vi "Query Chan Parameters (Input).vi"(7 "Channel (1: Chan A)":i32(ring)=1 items=["Channel A"=1, "Channel B"=2, "Channel C"=3, "Channel D"=4, "Channel E"=5, "Channel F"=6, "Channel G"=7, "Channel H"=8], 8 "error in (no error)":errorcluster, 11 "VISA resource name":refnum<visa-resource-name>) -> (0 "error out":errorcluster, 2 "Input Parameters":T1 {"Sync Source" items=["System (To)", "Channel A", "Channel B", "Channel C", "Channel D", "Channel E", "Channel F", "Channel G", "Channel H"]}, 3 "VISA resource name out":refnum<visa-resource-name>)   [LabVIEW 2012, in "Berkeley Nucleonics 500 Series.lvlib"]
doc: "This VI is used to read the input configuration of the selected channel."
uses:
  Berkeley Nucleonics 500 Series.lvlib
panel:
  # "The \"Gate Mode\" is currently only utilized by 9520/9530 instruments.  When controlling a 9520/9530,  the \"Gate Logic\" disabled setting is ignored."
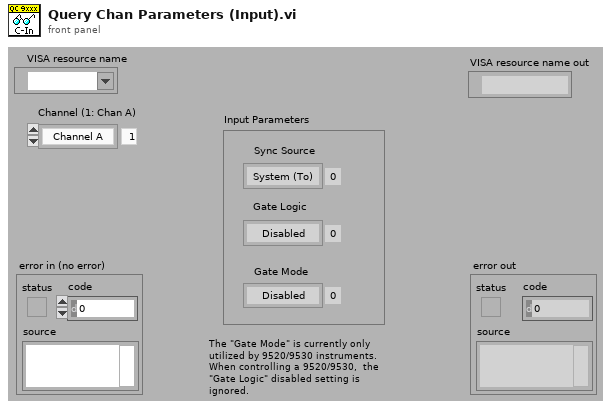
[diagram p1: front panel]
types:
  T1 = cluster{"Gate Logic":enum16{"Disabled", "Low", "High"}, "Sync Source":i32, "Gate Mode":enum16{"Disabled", "Pulse Inhibit", "Output Inhibit"}}
  T2 = enum16{"Disabled", "Pulse Inhibit", "Output Inhibit"}
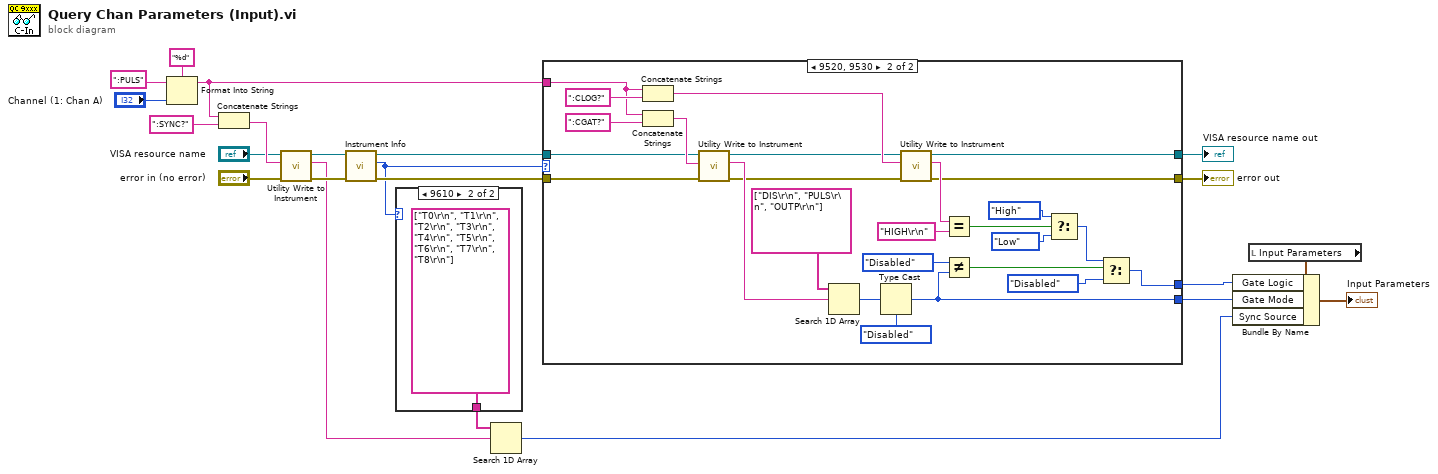
[diagram p0: block diagram]
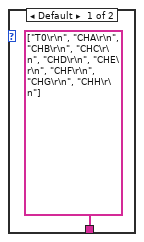
[diagram p2: hidden frame]
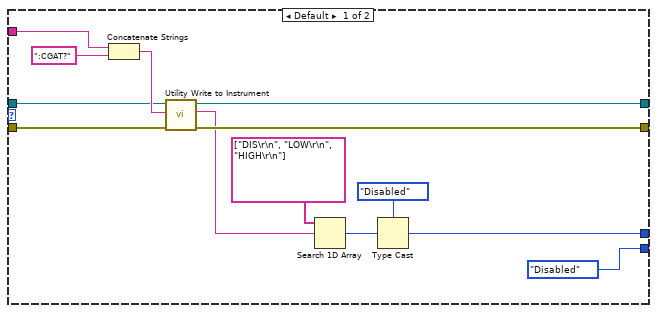
[diagram p3: hidden frame]
diagram:
  n1 = Format Into String(format string="%d", initial string=":PULS", "Channel (1: Chan A)") -> (resulting string=w5:string)  [unwired: 1 in, 1 out]
  n2 = Concatenate Strings(w5, ":SYNC?") -> (w10:string)
  n3 = call "Utility Write to Instrument.vi"("error in (no error)"="error in (no error)", "Write Buffer"=w10, "VISA resource name"="VISA resource name") -> ("error out"=w8:errorcluster, "Read Buffer"=w6:string, "VISA resource name out"=w7:refnum<visa-resource-name>)  [unwired: 6 out]
  n4 = call "Instrument Info.vi"("error in (no error)"=w8, "VISA resource name"=w7) -> ("error out"=w14:errorcluster, "Instr Model"=w1:u32, "VISA resource name out"=w13:refnum<visa-resource-name>)  [unwired: 7 out]
  n5 = case shown="9610" w1 {
    tunnel: [string[] ["T0\r\n", "CHA\r\n", "CHB\r\n", "CHC\r\n", "CHD\r\n", "CHE\r\n", "CHF\r\n", "CHG\r\n", "CHH\r\n"] string[] ["T0\r\n", "T1\r\n", "T2\r\n", "T3\r\n", "T4\r\n", "T5\r\n", "T6\r\n", "T7\r\n", "T8\r\n"]] -> w11
    frame Default {
    }
    frame 9610 {
    }
  }
  n6 = Search 1D Array(1D array=w11, element=w6) -> (index of element=w2:i32)  [unwired: 1 out]
  n7 = case shown="9520, 9530" w1 {
    tunnel: w5 -> [w36 w58]
    tunnel: w13 -> [w26 w53]
    tunnel: w14 -> [w27 w54]
    tunnel: [w34 w47] -> w19
    tunnel: [w33 w48] -> w18
    tunnel: [w30 w38] -> w15
    tunnel: [T2."Disabled" ("Gate Mode") w45] -> w12
    frame Default {
      n8 = Concatenate Strings(w36, ":CGAT?") -> (w35:string)
      n9 = call "Utility Write to Instrument.vi"("error in (no error)"=w27, "Write Buffer"=w35, "VISA resource name"=w26) -> ("error out"=w33:errorcluster, "Read Buffer"=w31:string, "VISA resource name out"=w34:refnum<visa-resource-name>)  [unwired: 6 out]
      n10 = Search 1D Array(1D array=string[] ["DIS\r\n", "LOW\r\n", "HIGH\r\n"], element=w31) -> (index of element=w29:i32)  [unwired: 1 out]
      n11 = Type Cast(type=enum16{"Disabled", "Low", "High"}."Disabled" ("Gate Logic"), x=w29) -> (*(type *) &x=w30:enum16{"Disabled", "Low", "High"})
    }
    frame 9520, 9530 {
      n12 = Concatenate Strings(w58, ":CLOG?") -> (w57:string)
      n13 = Concatenate Strings(w58, ":CGAT?") -> (w62:string)
      n14 = call "Utility Write to Instrument.vi"("error in (no error)"=w54, "Write Buffer"=w62, "VISA resource name"=w53) -> ("error out"=w52:errorcluster, "Read Buffer"=w60:string, "VISA resource name out"=w51:refnum<visa-resource-name>)  [unwired: 6 out]
      n15 = Search 1D Array(1D array=string[] ["DIS\r\n", "PULS\r\n", "OUTP\r\n"], element=w60) -> (index of element=w56:i32)  [unwired: 1 out]
      n16 = Type Cast(type=T2."Disabled" ("Gate Mode"), x=w56) -> (*(type *) &x=w45:T2)
      n17 = call "Utility Write to Instrument.vi"("error in (no error)"=w52, "Write Buffer"=w57, "VISA resource name"=w51) -> ("error out"=w48:errorcluster, "Read Buffer"=w50:string, "VISA resource name out"=w47:refnum<visa-resource-name>)  [unwired: 6 out]
      n18 = Equal?(x=w50, y="HIGH\r\n") -> (x = y?=w44:bool)
      n19 = Not Equal?(x=T2."Disabled" ("Gate Mode"), y=w45) -> (x != y?=w43:bool)
      n20 = Select(t=enum16{"Disabled", "Low", "High"}."High" ("Gate Logic"), s=w44, f=enum16{"Disabled", "Low", "High"}."Low" ("Gate Logic")) -> (s? t:f=w41:enum16{"Disabled", "Low", "High"})
      n21 = Select(t=w41, s=w43, f=enum16{"Disabled", "Low", "High"}."Disabled" ("Gate Logic")) -> (s? t:f=w38:enum16{"Disabled", "Low", "High"})
    }
  }
  "VISA resource name out" <- w19
  "error out" <- w18
  n22 = local read "Input Parameters"() -> (w16:T1)
  n23 = Bundle By Name(cluster=w16, "Gate Logic"=w15, "Gate Mode"=w12, "Sync Source"=w2) -> (→"Input Parameters":T1)
